vi "AlignReports.vi"(8 "error in (no error)":errorcluster, 10 "clPmuImpairRptArray":T1 {"Synx" format="%#_4g"}, 11 "clEvtReportArray":T1 {"Synx" format="%#_4g"}) -> (0 "error out":errorcluster, 2 "clPmuImpairRptArray":T1 {"Synx" format="%#_4g"}, 3 "clEvtReportArray":T1 {"Synx" format="%#_4g"})   [LabVIEW 2014, in "OutputToFilePlugins.lvlib" / "OutputToFileBasePlugin.lvclass"]
uses:
  OutputToFileBasePlugin.lvclass
  EventPlugins/EventPluginBaseClass/TypeDefs/clEvtReportArray.ctl
  EventPlugins/EventPluginBaseClass/TypeDefs/clEvtReport.ctl
  <vilib>/Utility/error.llb/Error Cluster From Error Code.vi
  <vilib>/ErrorRing/Error Ring.xnode
  EventPlugins/EventPluginBaseClass/EventPluginBaseClass.lvclass
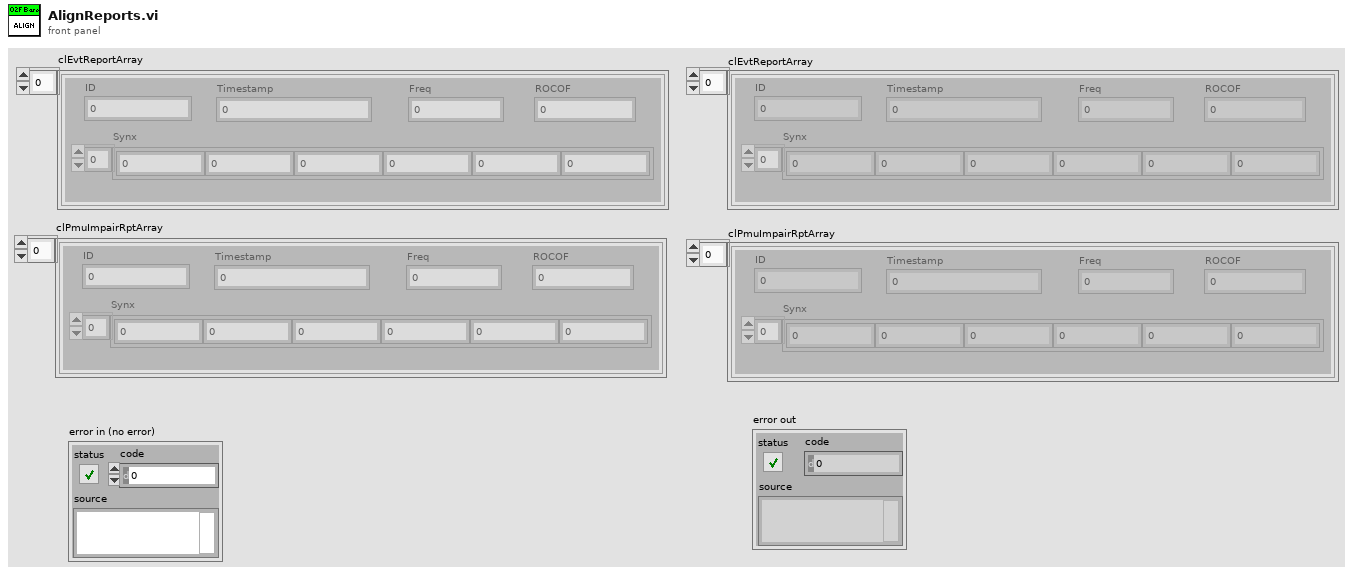
[diagram p1: front panel]
types:
  T1 = typedef "EventPlugins.lvlib/EventPluginBaseClass.lvclass/clEvtReportArray.ctl" = T2[]
  T2 = typedef "EventPlugins.lvlib/EventPluginBaseClass.lvclass/clEvtReport.ctl" = cluster{"Timestamp":dbl, "Synx":cdb[], "Freq":dbl, "ROCOF":dbl, "ID":i16}
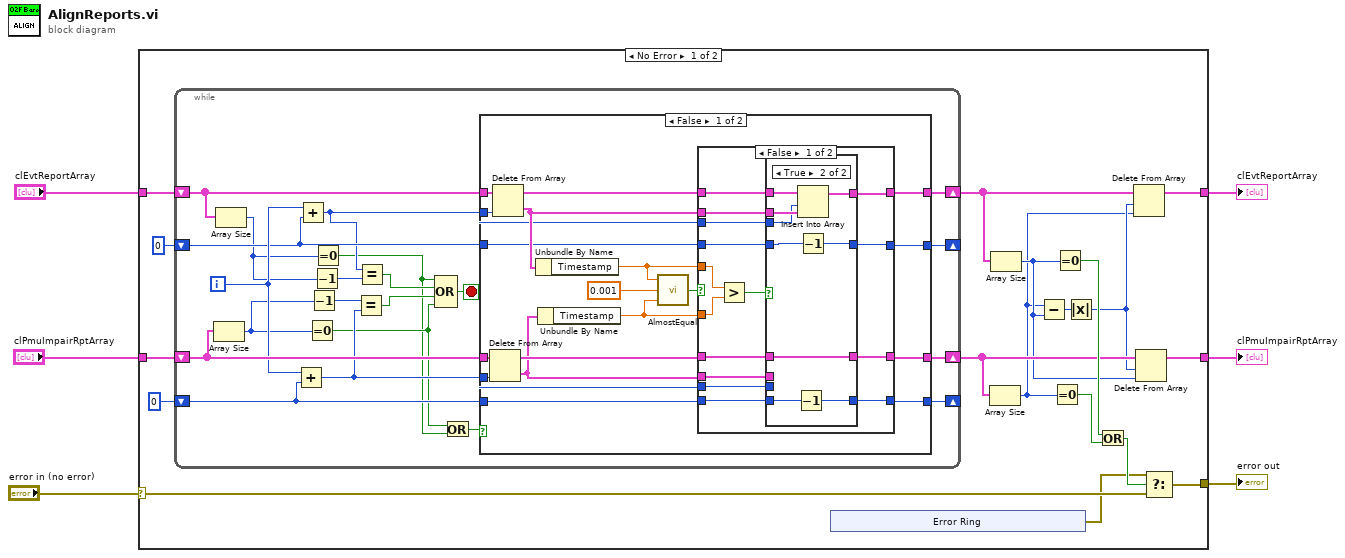
[diagram p0: block diagram]
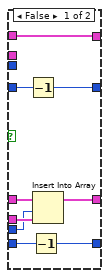
[diagram p2: hidden frame]
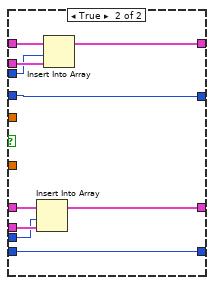
[diagram p3: hidden frame]
diagram:
  n1 = case shown="No Error" "error in (no error)" {
    selector: "error in (no error)" -> [w17 w116]
    tunnel: "clPmuImpairRptArray" -> [w24 _]
    tunnel: "clEvtReportArray" -> [w23 _]
    tunnel: [w9 _] -> w1
    tunnel: [w10 _] -> w2
    tunnel: [w15 w116] -> w3
    frame No Error {
      n2 = while {
        shift-right: [w50] -> w14
        shift-left: w23 -> [w46]
        shift-right: [w49] -> w13
        shift-left: w24 -> [w45]
        shift-right: [w47] -> _
        shift-left: 0 -> [w40]
        shift-right: [w48] -> _
        shift-left: 0 -> [w39]
        i -> [w44]
        stop <- w41 stop-if-true
        n3 = Array Size(array=w45) -> (size(s)=w35:i32)
        n4 = Array Size(array=w46) -> (size(s)=w33:i32)
        n5 = Add(x=w44, y=w39) -> (x+y=w37:i32)
        n6 = Add(x=w44, y=w40) -> (x+y=w38:i32)
        n7 = Equal To 0?(x=w35) -> (x = 0?=w31:bool)
        n8 = Decrement(x=w35) -> (x-1=w36:i32)
        n9 = Decrement(x=w33) -> (x-1=w34:i32)
        n10 = Equal To 0?(x=w33) -> (x = 0?=w30:bool)
        n11 = Equal?(x=w36, y=w37) -> (x = y?=w43:bool)
        n12 = Equal?(x=w38, y=w34) -> (x = y?=w42:bool)
        n13 = Compound Arithmetic op=OR(w30, w42, w43, w31) -> (w41:bool)
        n14 = Or(x=w31, y=w30) -> (x .or. y?=w32:bool)
        n15 = case shown="False" w32 {
          tunnel: [w64 w115] -> w50
          tunnel: [w63 w113] -> w49
          tunnel: [w62 w112] -> w48
          tunnel: [w61 w114] -> w47
          tunnel: w46 -> [w60 w115]
          tunnel: w45 -> [w59 w113]
          tunnel: w40 -> [w58 w114]
          tunnel: w39 -> [w57 w112]
          tunnel: w38 -> [w56 _]
          tunnel: w37 -> [w55 _]
          frame False {
            n16 = Delete From Array(array=w59, index=w55) -> (deleted portion=w65:T2, array with subset deleted=w66:T1)  [unwired: 1 in]
            n17 = Delete From Array(array=w60, index=w56) -> (deleted portion=w67:T2, array with subset deleted=w68:T1)  [unwired: 1 in]
            n18 = Unbundle By Name(w67) -> ("Timestamp"=w52:dbl)
            n19 = Unbundle By Name(w65) -> ("Timestamp"=w53:dbl)
            n20 = call "AlmostEqual.vi"("Y"=w53, "Tolerance (0.01)"=0.001, "X"=w52) -> ("X = Y"=w54:bool)
            n21 = case shown="False" w54 {
              tunnel: w68 -> [w81 w111]
              tunnel: w67 -> [w80 w110]
              tunnel: w58 -> [w79 w104]
              tunnel: w66 -> [w74 w109]
              tunnel: w65 -> [w73 w108]
              tunnel: w57 -> [w77 w105]
              tunnel: [w75 w107] -> w64
              tunnel: [w71 w106] -> w63
              tunnel: [w76 w105] -> w62
              tunnel: [w72 w104] -> w61
              tunnel: w52 -> [w83 _]
              tunnel: w53 -> [w82 _]
              tunnel: w56 -> [w70 w103]
              tunnel: w55 -> [w69 w102]
              frame False {
                n22 = Greater?(x=w83, y=w82) -> (0:w78:bool)
                n23 = case shown="True" w78 {
                  tunnel: w81 -> [w90 w101]
                  tunnel: w80 -> [_ w100]
                  tunnel: w79 -> [w87 w97]
                  tunnel: w77 -> [w89 w95]
                  tunnel: [w86 w93] -> w76
                  tunnel: [w90 w99] -> w75
                  tunnel: w74 -> [w92 w98]
                  tunnel: w73 -> [w91 _]
                  tunnel: [w85 w96] -> w72
                  tunnel: [w88 w98] -> w71
                  tunnel: w70 -> [_ w94]
                  tunnel: w69 -> [w84 _]
                  frame False {
                    n24 = Decrement(x=w87) -> (x-1=w85:i32)
                    n25 = Decrement(x=w89) -> (x-1=w86:i32)
                    n26 = Insert Into Array(array=w92, index=w84, new element=w91) -> (w88:T1)
                  }
                  frame True {
                    n27 = Decrement(x=w95) -> (x-1=w93:i32)
                    n28 = Insert Into Array(array=w101, index=w94, new element=w100) -> (w99:T1)
                    n29 = Decrement(x=w97) -> (x-1=w96:i32)
                  }
                }
              }
              frame True {
                n30 = Insert Into Array(array=w109, index=w102, new element=w108) -> (w106:T1)
                n31 = Insert Into Array(array=w111, index=w103, new element=w110) -> (w107:T1)
              }
            }
          }
          frame True {
          }
        }
      }
      n32 = xnode "Error Ring"() -> ("error out"=w16:errorcluster)
      n33 = Array Size(array=w13) -> (size(s)=w7:i32)
      n34 = Array Size(array=w14) -> (size(s)=w8:i32)
      n35 = Subtract(x=w7, y=w8) -> (x-y=w12:i32)
      n36 = Equal To 0?(x=w7) -> (x = 0?=w18:bool)
      n37 = Equal To 0?(x=w8) -> (x = 0?=w19:bool)
      n38 = Absolute Value(x=w12) -> (abs(x)=w11:i32)
      n39 = Or(x=w19, y=w18) -> (x .or. y?=w20:bool)
      n40 = Delete From Array(array=w14, length=w11, index=w7) -> (array with subset deleted=w10:T1)  [unwired: 1 out]
      n41 = Delete From Array(array=w13, length=w11, index=w8) -> (array with subset deleted=w9:T1)  [unwired: 1 out]
      n42 = Select(t=w16, s=w20, f=w17) -> (s? t:f=w15:errorcluster)
    }
    frame Error {
    }
  }
  "error out" <- w3
  "clEvtReportArray" <- w2
  "clPmuImpairRptArray" <- w1
